vi "parse_to_rio.vi"(4 "error in":errorcluster, 7 "msg in":string) -> (0 "error out":errorcluster, 2 "to_rio":T1, 3 "msg out":string)   [LabVIEW 2016]
uses:
  <userlib>/ROS for LabVIEW Software/ROS/MessageParsing/std_msgs/subs/parse_float64_scalar.vi
  <userlib>/ROS for LabVIEW Software/ROS/MessageParsing/std_msgs/subs/parse_i8_scalar.vi
  <userlib>/ROS for LabVIEW Software/ROS/MessageParsing/std_msgs/subs/parse_time_scalar.vi
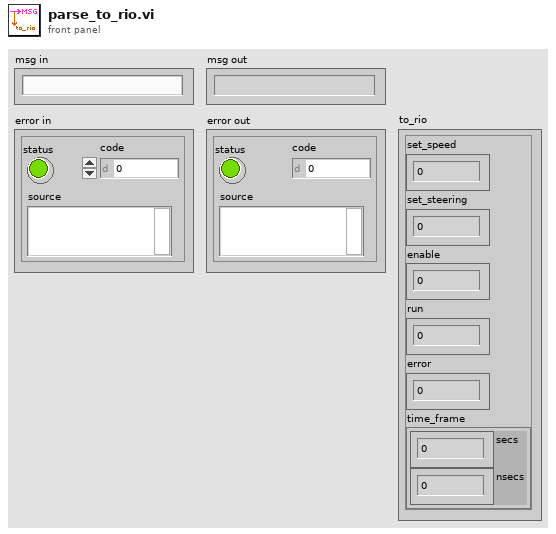
[diagram p1: front panel]
types:
  T1 = cluster{"set_speed":dbl, "set_steering":dbl, "enable":i8, "run":i8, "error":i8, "time_frame":cluster{"secs":i32, "nsecs":i32}}
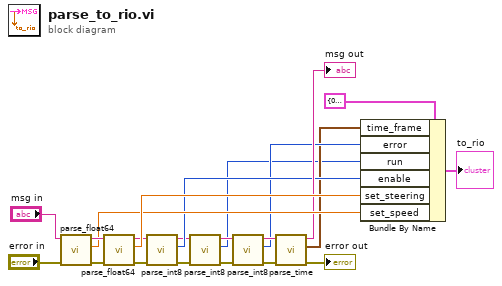
[diagram p0: block diagram]
diagram:
  n1 = call-poly <userlib>:"parse_float64.vi"("error in"="error in", "msg in"="msg in") -> ("error out"=w20:errorcluster, "number"=w17:dbl, "msg out"=w19:string)  [unwired: 3 in]
  n2 = call-poly <userlib>:"parse_float64.vi"("error in"=w20, "msg in"=w19) -> ("error out"=w15:errorcluster, "number"=w18:dbl, "msg out"=w16:string)  [unwired: 3 in]
  n3 = call-poly <userlib>:"parse_int8.vi"("error in"=w15, "msg in"=w16) -> ("error out"=w12:errorcluster, "number"=w11:i8, "msg out"=w10:string)  [unwired: 3 in]
  n4 = call-poly <userlib>:"parse_int8.vi"("error in"=w12, "msg in"=w10) -> ("error out"=w7:errorcluster, "number"=w1:i8, "msg out"=w6:string)  [unwired: 3 in]
  n5 = call-poly <userlib>:"parse_int8.vi"("error in"=w7, "msg in"=w6) -> ("error out"=w9:errorcluster, "number"=w3:i8, "msg out"=w8:string)  [unwired: 3 in]
  n6 = call-poly <userlib>:"parse_time.vi"("error in"=w9, "msg in"=w8) -> ("error out"=→"error out":errorcluster, "Time"=w2:cluster{"secs":i32, "nsecs":i32}, "msg out"=→"msg out":string)  [unwired: 3 in]
  n7 = Bundle By Name(cluster=T1 {"set_speed"=0.0, "set_steering"=0.0, "enable"=0, "run"=0, "error"=0, "time_frame"={"secs"=0, "nsecs"=0}} ("to_rio"), "time_frame"=w2, "error"=w3, "run"=w1, "enable"=w11, "set_steering"=w18, "set_speed"=w17) -> (→"to_rio":T1)
